vi "Get Rect.vi"(4 "y":sgl, 5 "x":sgl, 6 "Height":i16, 7 "Width":i16) -> (0 "Bottom":sgl, 1 "Right":sgl, 2 "Top":sgl, 3 "Left":sgl)   [LabVIEW 2022 SP3, in "RectangleShape.lvclass"]
uses:
  RectangleShape.lvclass
  RectangleShape.lvclass/RectangleShape.ctl
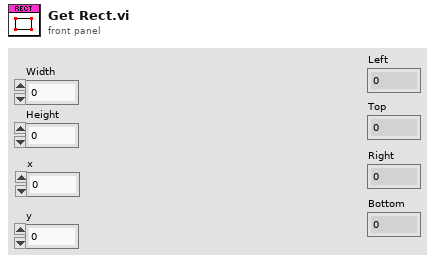
[diagram p1: front panel]
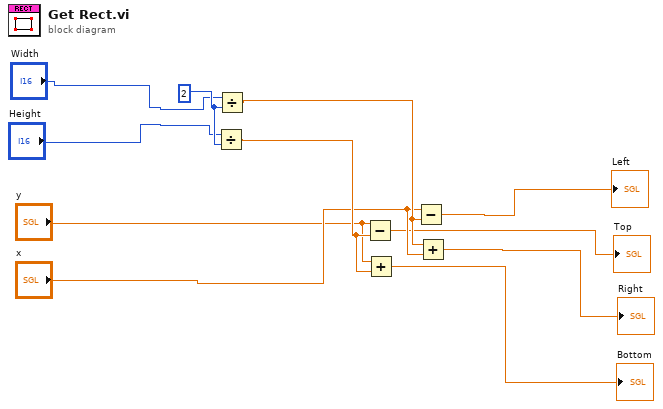
[diagram p0: block diagram]
diagram:
  w11 = 2
  n1 = Divide(x="Height", y=w11) -> (x/y=w9:dbl)
  n2 = Divide(x="Width", y=w11) -> (x/y=w10:dbl)
  n3 = Subtract(x="y", y=w9) -> (x-y=→"Top":dbl)
  n4 = Add(x="y", y=w9) -> (x+y=→"Bottom":dbl)
  n5 = Subtract(x="x", y=w10) -> (x-y=→"Left":dbl)
  n6 = Add(x=w10, y="x") -> (x+y=→"Right":dbl)
